vi "4-libssh2_sftp_read-binary data truncated.vi"() -> ()   [LabVIEW 2013, in "libssh2_integration_tests.lvlib"]
uses:
  libssh2_integration_tests.lvlib
  libssh2/libssh2.lvlib
  <vilib>/addons/_JKI Toolkits/Caraya/classes/Test/Test.lvclass
  <vilib>/addons/_JKI Toolkits/Caraya/classes/Assert/Assert.lvclass
panel:
  out "error out":errorcluster
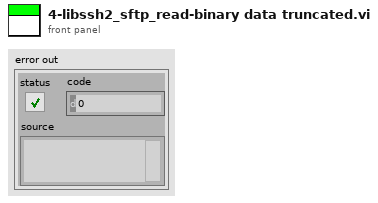
[diagram p1: front panel]
types:
  T1 = typedef "libssh2.lvlib/Session Refnum.ctl" = refnum<k1>
  T2 = typedef "libssh2.lvlib/SFTP Refnum.ctl" = refnum<k1>
  T3 = typedef "libssh2.lvlib/SFTP Handle Refnum.ctl" = refnum<k1>
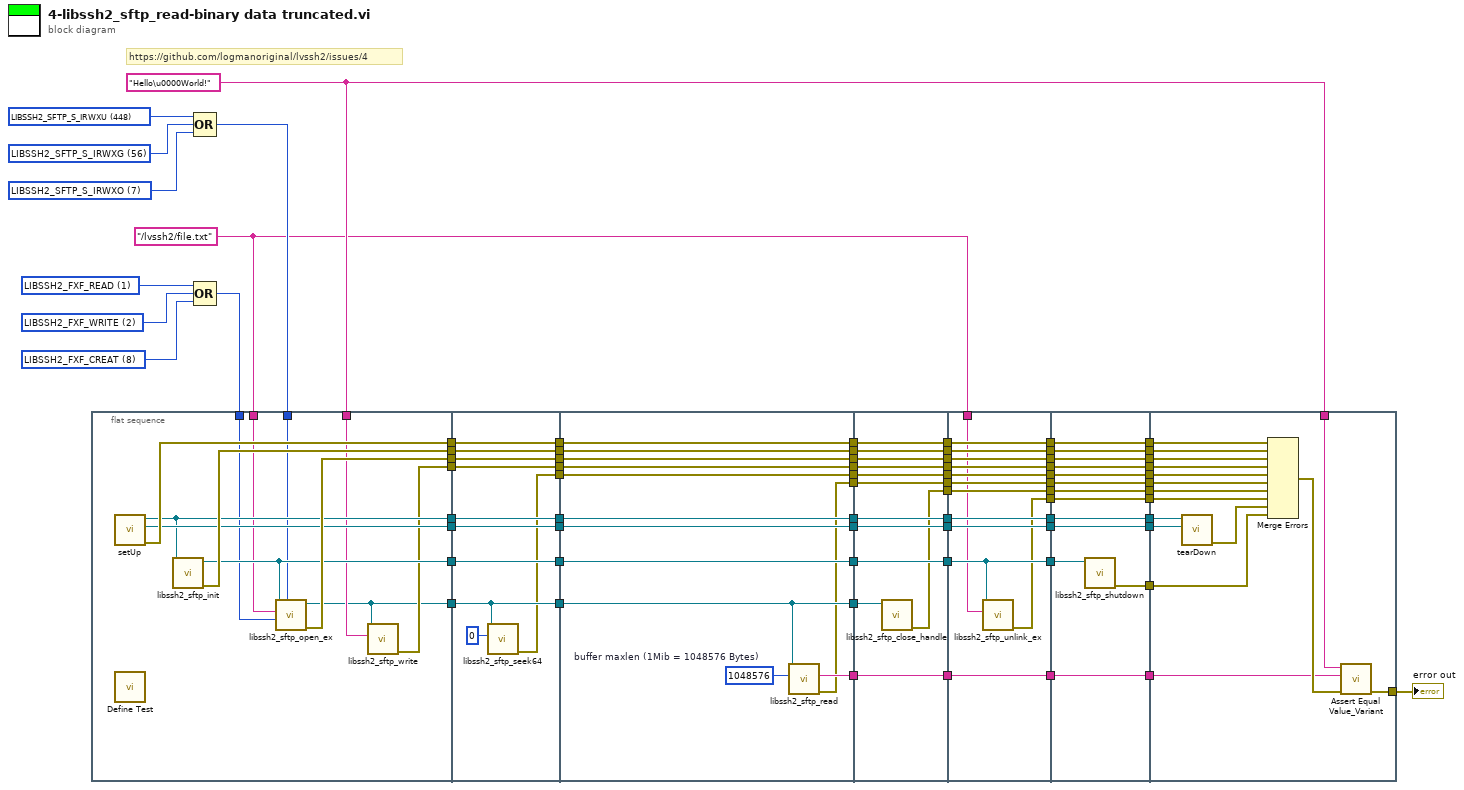
[diagram p0: block diagram]
diagram:
  w2 = "Hello\u0000World!" ("buffer")
  w5 = u32 2 items=["LIBSSH2_FXF_READ"=1, "LIBSSH2_FXF_WRITE"=2, "LIBSSH2_FXF_APPEND"=4, "LIBSSH2_FXF_CREAT"=8, "LIBSSH2_FXF_TRUNC"=16, "LIBSSH2_FXF_EXCL"=32] ("flags")
  w6 = u32 1 items=["LIBSSH2_FXF_READ"=1, "LIBSSH2_FXF_WRITE"=2, "LIBSSH2_FXF_APPEND"=4, "LIBSSH2_FXF_CREAT"=8, "LIBSSH2_FXF_TRUNC"=16, "LIBSSH2_FXF_EXCL"=32] ("flags")
  w4 = u32 8 items=["LIBSSH2_FXF_READ"=1, "LIBSSH2_FXF_WRITE"=2, "LIBSSH2_FXF_APPEND"=4, "LIBSSH2_FXF_CREAT"=8, "LIBSSH2_FXF_TRUNC"=16, "LIBSSH2_FXF_EXCL"=32] ("flags")
  w1 = "/lvssh2/file.txt" ("filename")
  w8 = 7 items=["LIBSSH2_SFTP_S_IRWXU"=448, "LIBSSH2_SFTP_S_IRUSR"=256, "LIBSSH2_SFTP_S_IWUSR"=128, "LIBSSH2_SFTP_S_IXUSR"=64, "LIBSSH2_SFTP_S_IRWXG"=56, "LIBSSH2_SFTP_S_IRGRP"=32, "LIBSSH2_SFTP_S_IWGRP"=16, "LIBSSH2_SFTP_S_IXGRP"=8, "LIBSSH2_SFTP_S_IRWXO"=7, "LIBSSH2_SFTP_S_IROTH"=4, "LIBSSH2_SFTP_S_IWOTH"=2, "LIBSSH2_SFTP_S_IXOTH"=1] ("mode")
  w9 = 56 items=["LIBSSH2_SFTP_S_IRWXU"=448, "LIBSSH2_SFTP_S_IRUSR"=256, "LIBSSH2_SFTP_S_IWUSR"=128, "LIBSSH2_SFTP_S_IXUSR"=64, "LIBSSH2_SFTP_S_IRWXG"=56, "LIBSSH2_SFTP_S_IRGRP"=32, "LIBSSH2_SFTP_S_IWGRP"=16, "LIBSSH2_SFTP_S_IXGRP"=8, "LIBSSH2_SFTP_S_IRWXO"=7, "LIBSSH2_SFTP_S_IROTH"=4, "LIBSSH2_SFTP_S_IWOTH"=2, "LIBSSH2_SFTP_S_IXOTH"=1] ("mode")
  w10 = 448 items=["LIBSSH2_SFTP_S_IRWXU"=448, "LIBSSH2_SFTP_S_IRUSR"=256, "LIBSSH2_SFTP_S_IWUSR"=128, "LIBSSH2_SFTP_S_IXUSR"=64, "LIBSSH2_SFTP_S_IRWXG"=56, "LIBSSH2_SFTP_S_IRGRP"=32, "LIBSSH2_SFTP_S_IWGRP"=16, "LIBSSH2_SFTP_S_IXGRP"=8, "LIBSSH2_SFTP_S_IRWXO"=7, "LIBSSH2_SFTP_S_IROTH"=4, "LIBSSH2_SFTP_S_IWOTH"=2, "LIBSSH2_SFTP_S_IXOTH"=1] ("mode")
  # "https://github.com/logmanoriginal/lvssh2/issues/4"
  n1 = flat-sequence {
    tunnel: [w86] -> w74
    tunnel: [w85] -> w73
    tunnel: [w84] -> w72
    tunnel: [w83] -> w71
    tunnel: [w82] -> w70
    tunnel: [w81] -> w69
    tunnel: [w75] -> w68
    tunnel: w2 -> [w80]
    tunnel: [w79] -> w67
    tunnel: w3 -> [w76]
    tunnel: w1 -> [w77]
    tunnel: w7 -> [w78]
    tunnel: w74 -> [w96]
    tunnel: [w96] -> w66
    tunnel: w73 -> [w95]
    tunnel: [w95] -> w65
    tunnel: w72 -> [w94]
    tunnel: [w94] -> w64
    tunnel: w71 -> [w93]
    tunnel: [w93] -> w63
    tunnel: w70 -> [w92]
    tunnel: [w92] -> w62
    tunnel: w69 -> [w91]
    tunnel: [w91] -> w61
    tunnel: w68 -> [w89]
    tunnel: [w89] -> w60
    tunnel: w67 -> [w90]
    tunnel: [w90] -> w59
    tunnel: [w88] -> w58
    tunnel: w66 -> [w108]
    tunnel: [w108] -> w57
    tunnel: w65 -> [w107]
    tunnel: [w107] -> w56
    tunnel: w64 -> [w106]
    tunnel: [w106] -> w55
    tunnel: w63 -> [w105]
    tunnel: [w105] -> w54
    tunnel: w62 -> [w104]
    tunnel: [w104] -> w53
    tunnel: w61 -> [w103]
    tunnel: [w103] -> w52
    tunnel: w60 -> [w100]
    tunnel: [w100] -> w51
    tunnel: w59 -> [w102]
    tunnel: [w102] -> w50
    tunnel: [w99] -> w49
    tunnel: [w98] -> w48
    tunnel: w58 -> [w97]
    tunnel: [w97] -> w47
    tunnel: [w114] -> w40
    tunnel: w57 -> [w120]
    tunnel: [w120] -> w41
    tunnel: w56 -> [w119]
    tunnel: [w119] -> w42
    tunnel: w55 -> [w118]
    tunnel: [w118] -> w43
    tunnel: w54 -> [w117]
    tunnel: [w117] -> w44
    tunnel: w53 -> [w116]
    tunnel: [w116] -> w45
    tunnel: w52 -> [w115]
    tunnel: [w115] -> w46
    tunnel: w51 -> [w113]
    tunnel: w50 -> [w112]
    tunnel: [w112] -> w39
    tunnel: [w111] -> w38
    tunnel: w49 -> [w111]
    tunnel: [w110] -> w37
    tunnel: w48 -> [w110]
    tunnel: w47 -> [w109]
    tunnel: [w109] -> w36
    tunnel: w46 -> [w133]
    tunnel: [w133] -> w35
    tunnel: w45 -> [w132]
    tunnel: [w132] -> w34
    tunnel: w44 -> [w123]
    tunnel: [w123] -> w33
    tunnel: w43 -> [w131]
    tunnel: [w131] -> w32
    tunnel: w42 -> [w130]
    tunnel: [w130] -> w31
    tunnel: w41 -> [w129]
    tunnel: [w129] -> w30
    tunnel: w40 -> [w128]
    tunnel: [w128] -> w29
    tunnel: w39 -> [w127]
    tunnel: [w127] -> w28
    tunnel: w38 -> [w126]
    tunnel: [w126] -> w27
    tunnel: w37 -> [w125]
    tunnel: [w125] -> w26
    tunnel: w36 -> [w124]
    tunnel: [w124] -> w25
    tunnel: w1 -> [w122]
    tunnel: [w121] -> w24
    tunnel: w35 -> [w146]
    tunnel: [w146] -> w23
    tunnel: w34 -> [w145]
    tunnel: [w145] -> w22
    tunnel: w33 -> [w142]
    tunnel: w32 -> [w144]
    tunnel: [w144] -> w21
    tunnel: w31 -> [w143]
    tunnel: [w143] -> w20
    tunnel: [w141] -> w19
    tunnel: w30 -> [w140]
    tunnel: [w140] -> w18
    tunnel: [w139] -> w17
    tunnel: w29 -> [w139]
    tunnel: w28 -> [w138]
    tunnel: [w138] -> w16
    tunnel: [w137] -> w15
    tunnel: w27 -> [w137]
    tunnel: [w136] -> w14
    tunnel: w26 -> [w136]
    tunnel: w25 -> [w135]
    tunnel: [w135] -> w13
    tunnel: w24 -> [w134]
    tunnel: [w134] -> w12
    tunnel: w23 -> [w162]
    tunnel: w22 -> [w161]
    tunnel: w21 -> [w160]
    tunnel: [w157] -> w11
    tunnel: w20 -> [w156]
    tunnel: w19 -> [w155]
    tunnel: w18 -> [w154]
    tunnel: w17 -> [w153]
    tunnel: w16 -> [w152]
    tunnel: w15 -> [w151]
    tunnel: w14 -> [w150]
    tunnel: w2 -> [w149]
    tunnel: w13 -> [w148]
    tunnel: w12 -> [w147]
    frame #0 {
      n2 = call "setUp.vi"() -> ("error out"=w84:errorcluster, "connection ID"=w82:refnum<k5>, "session"=w81:T1)  [unwired: 9 in]
      n3 = call <vilib>:"Define Test.vi"() -> ()  [unwired: 10 in, 2 out]
      n4 = call "libssh2_sftp_init.vi"("session"=w81) -> ("error out"=w85:errorcluster, "sftp"=w83:T2)  [unwired: 9 in]
      n5 = call "libssh2_sftp_open_ex.vi"("mode"=w78, "flags"=w76, "filename"=w77, "sftp"=w83) -> ("error out"=w86:errorcluster, "sftp handle"=w75:T3)  [unwired: 6 in]
      n6 = call "libssh2_sftp_write.vi"("buffer"=w80, "sftp handle"=w75) -> ("error out"=w79:errorcluster)  [unwired: 8 in, 1 out]
    }
    frame #1 {
      n7 = call "libssh2_sftp_seek64.vi"("offset"=u64 0, "sftp handle"=w89) -> ("error out"=w88:errorcluster)  [unwired: 9 in]
    }
    frame #2 {
      w101 = 1048576  # buffer maxlen (1Mib = 1048576 Bytes)
      n8 = call "libssh2_sftp_read.vi"("buffer maxlen"=w101, "sftp handle"=w100) -> ("error out"=w98:errorcluster, "buffer"=w99:string)  [unwired: 7 in, 1 out]
    }
    frame #3 {
      n9 = call "libssh2_sftp_close_handle.vi"("sftp handle"=w113) -> ("error out"=w114:errorcluster)  [unwired: 10 in]
    }
    frame #4 {
      n10 = call "libssh2_sftp_unlink_ex.vi"("file"=w122, "sftp"=w123) -> ("error out"=w121:errorcluster)  [unwired: 9 in]
    }
    frame #5 {
      n11 = call "libssh2_sftp_shutdown.vi"("sftp"=w142) -> ("error out"=w141:errorcluster)  [unwired: 10 in]
    }
    frame #6 {
      n12 = call "tearDown.vi"("connection ID"=w161, "session"=w162) -> ("error out"=w159:errorcluster)  [unwired: 9 in]
      n13 = Merge Errors(w160, w156, w154, w152, w148, w150, w153, w147, w159, w155) -> (w158:errorcluster)
      n14 = call <vilib>:"Assert Equal Value_Variant.vi"("error in (no error)"=w158, "Y"=w151, "X"=w149) -> ("error out"=w157:errorcluster)  [unwired: 7 in, 1 out]
    }
  }
  n15 = Compound Arithmetic op=OR(w10, w9, w8) -> (w7:i32)
  n16 = Compound Arithmetic op=OR(w6, w5, w4) -> (w3:u32)
  "error out" <- w11
